vi "Ionpump.vi"() -> (0 "Saes Error":errorcluster, 1 "output 1":dbl, 2 "Ion\nPump":string="0 nA")   [LabVIEW 2014]
uses:
  <vilib>/Instr/_visa.llb/VISA Configure Serial Port (Instr).vi
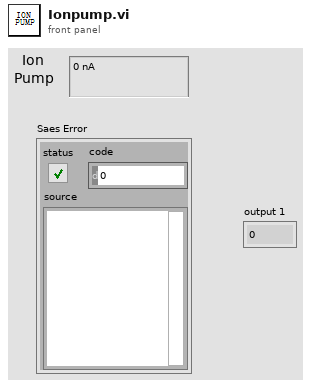
[diagram p1: front panel]
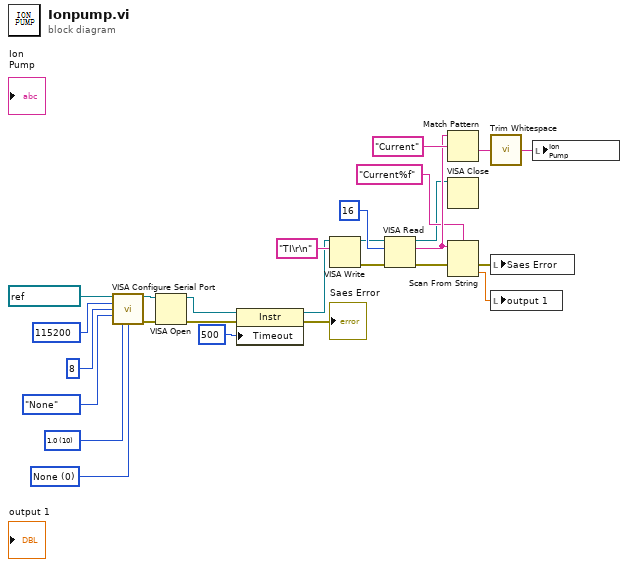
[diagram p0: block diagram]
diagram:
  w10 = u16 0 items=["None", "XON/XOFF", "RTS/CTS", "XON/XOFF & RTS/CTS", "DTR/DSR", "XON/XOFF & DTR/DSR"] ("flow control (0:none)")
  w11 = u16 10 items=["1.0"=10, "1.5"=15, "2.0"=20] ("stop bits (10: 1 bit)")
  n1 = call-poly "VISA Configure Serial Port"("VISA resource name"=refnum<visa-resource-name> "COM17", "baud rate (9600)"=u32 115200, "data bits (8)"=u16 8, "parity (0:none)"=enum16{"None", "Odd", "Even", "Mark", "Space"}."None", "stop bits (10: 1 bit)"=w11, "flow control (0:none)"=w10) -> ("VISA resource name out"=w15:refnum<visa-resource-name>, "error out"=w5:errorcluster)  [unwired: 8 in]
  n2 = VISA Open(error in (no error)=w5, VISA resource name=w15) -> (VISA resource name=w7:refnum<visa-resource-name>, error out=w4:errorcluster)  [unwired: 3 in]
  n3 = property class="Instr"(reference=w7, error in=w4, "Timeout"=500) -> (reference out=w3:refnum<visa-resource-name>, error out=→"Saes Error":errorcluster)
  n4 = VISA Write(VISA resource name=w3, write buffer="TI\r\n") -> (VISA resource name out=w16:refnum<visa-resource-name>, error out=w2:errorcluster)  [unwired: 1 in, 1 out]
  n5 = VISA Read(VISA resource name=w16, byte count=u32 16, error in (no error)=w2) -> (VISA resource name out=w1:refnum<visa-resource-name>, read buffer=w20:string, error out=w24:errorcluster)  [unwired: 1 out]
  n6 = Match Pattern(string=w20, regular expression="Current") -> (after substring=w22:string)  [unwired: 1 in, 3 out]
  n7 = VISA Close(VISA resource name=w1) -> ()  [unwired: 1 in, 1 out]
  n8 = Scan From String(format string="Current%f" ("regular expression"), input string=w20, error in=w24) -> (error out=w25:errorcluster, output 1=w26:dbl)  [unwired: 2 in, 2 out]
  n9 = call <vilib>:"Trim Whitespace.vi"("string"=w22) -> ("trimmed string"=w23:string)  [unwired: 1 in]
  n10 = local write "Saes Error"(w25) -> ()
  n11 = local write "output 1"(w26) -> ()
  n12 = local write "Ion\nPump"(w23) -> ()
